vi "GetPicture.vi"() -> ()   [LabVIEW 2013]
panel:
  in  "GetPicture":bool
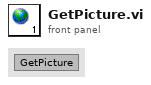
[diagram p1: front panel]
diagram:
